vi "ROS_Write_Motors.vi"(7 "SP_V_in":T1={"topic port"=0, "Node"="", "topic"="", "type"="", "node port"=0, "error "={"status"=FALSE, "code"=0, "source"=""}, "Direction"=enum."Node", "Update (ms)"=1, "FIFO size"=1}, 8 "error in (no error)":errorcluster, 9 "W_in":sgl, 10 "V_in":sgl, 11 "SP_W_in":T1={"topic port"=0, "Node"="", "topic"="", "type"="", "node port"=0, "error "={"status"=FALSE, "code"=0, "source"=""}, "Direction"=enum."Node", "Update (ms)"=1, "FIFO size"=1}) -> (0 "error out":errorcluster, 3 "SP_W_out":T1={"topic port"=0, "Node"="", "topic"="", "type"="", "node port"=0, "error "={"status"=FALSE, "code"=0, "source"=""}, "Direction"=enum."Node", "Update (ms)"=1, "FIFO size"=1}, 5 "SP_V_out":T1={"topic port"=0, "Node"="", "topic"="", "type"="", "node port"=0, "error "={"status"=FALSE, "code"=0, "source"=""}, "Direction"=enum."Node", "Update (ms)"=1, "FIFO size"=1})   [LabVIEW 2017]
doc: "Write robot's forward velocity V and rotation velocity w to ROS motors' topics"
uses:
  <vilib>/Tufts CEEO ROS for LabVIEW Software/ROS/Code/SubVIs/_ROSControl.ctl
  <vilib>/Tufts CEEO ROS for LabVIEW Software/ROS/Code/SubVIs/_ROSDirection.ctl
  <vilib>/Tufts CEEO ROS for LabVIEW Software/ROS/MessageBuilding/std_msgs/subs/float32Scalar.vi
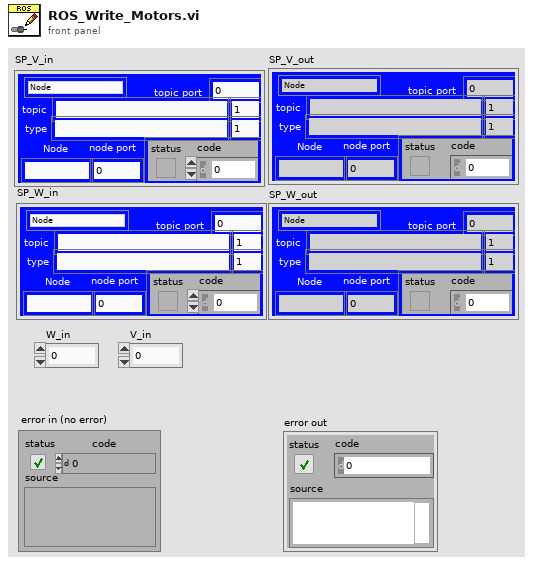
[diagram p1: front panel]
types:
  T1 = typedef "_ROSControl.ctl" = cluster{"topic port":u16, "Node":string, "topic":string, "type":string, "node port":u16, "error ":errorcluster, "Direction":T2, "Update (ms)":u16, "FIFO size":u16}
  T2 = typedef "_ROSDirection.ctl" = enum16{"Node", "Publisher", "Subscriber", "ServiceClient", "ServiceProvider"}
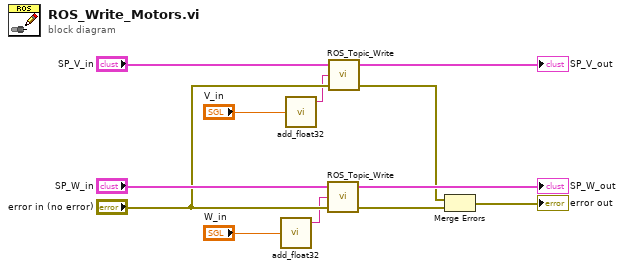
[diagram p0: block diagram]
diagram:
  n1 = call-poly <vilib>:"add_float32.vi"("Numeric"="W_in") -> ("msg out"=w1:string)  [unwired: 4 in]
  n2 = call-poly <vilib>:"add_float32.vi"("Numeric"="V_in") -> ("msg out"=w2:string)  [unwired: 4 in]
  n3 = call <vilib>:"ROS_Topic_Write.vi"("error in (no error)"="error in (no error)", "Msg in"=w1, "ROS in"="SP_W_in") -> ("error out"=w6:errorcluster, "ROS out"=→"SP_W_out":T1)  [unwired: 1 in]
  n4 = call <vilib>:"ROS_Topic_Write.vi"("error in (no error)"="error in (no error)", "Msg in"=w2, "ROS in"="SP_V_in") -> ("error out"=w5:errorcluster, "ROS out"=→"SP_V_out":T1)  [unwired: 1 in]
  n5 = Merge Errors(w5, w6) -> (→"error out":errorcluster)
